vi "Suppress Error.vi"(6 "Error Code":i32, 7 "Error In":errorcluster) -> (2 "Error Supressed?":bool, 3 "Error Out":errorcluster)   [LabVIEW 2020, in "Configit.lvlib"]
uses:
  Configit.lvlib
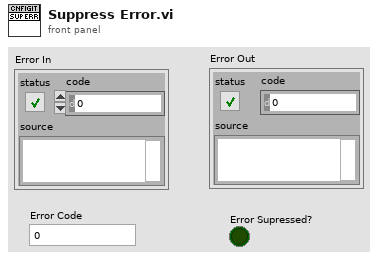
[diagram p1: front panel]
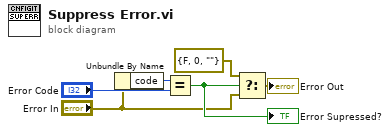
[diagram p0: block diagram]
diagram:
  n1 = Unbundle By Name("Error In") -> ("code"=w3:i32)
  n2 = Equal?(x=w3, y="Error Code") -> (x = y?=w5:bool)
  "Error Supressed?" <- w5
  n3 = Select(t=errorcluster {"status"=FALSE, "code"=0, "source"=""} ("error IO"), s=w5, f="Error In") -> (s? t:f=→"Error Out":errorcluster)
